vi "IRH3T.vi"(8 "Due Dates":u16[](array[numeric]), 9 "Initial Tardiness":i32, 10 "Schedule 2B Improved":u16[](array[numeric]), 11 "Proocessing Times  (Machines x Jobs)":u16[][](array[numeric])=[[208, 80, 8, 184, 218, 197, 100, 5], [64, 30, 39, 91, 257, 38, 34, 447], [23, 215, 125, 135, 165, 136, 164, 37], [88, 22, 207, 5, 58, 213, 52, 355], [6, 181, 111, 222, 27, 259, 91, 103], [149, 37, 22, 14, 71, 155, 536, 16], [113, 71, 274, 348, 187, 1, 3, 3], [349, 364, 214, 1, 17, 1, 20, 34]]) -> (2 "Total Tardiness":i32, 3 "IRH3T (Reordered) Schedule Out":u16[](array[numeric]))   [LabVIEW 2013]
uses:
  Classes/GanntChart_Class/Operation to Machine Job Tuple.vi
  Classes/GanntChart.lvclass
panel:
  out "IRH3T Schedule Out":u16[](array[numeric])
  out "String":string="Total Tardiness has been improved. Total Tardiness is now %d"
  out "Job Completion Times":u16[](array[numeric])
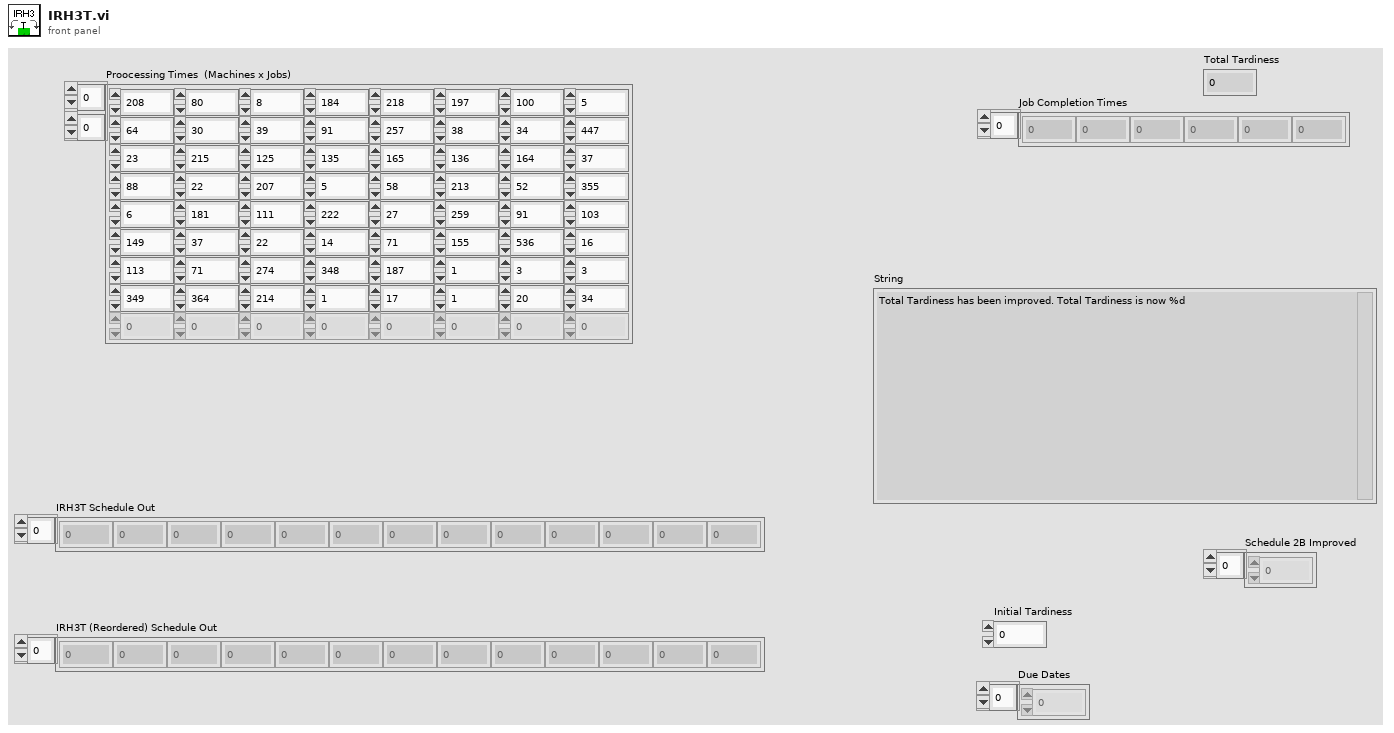
[diagram p1: front panel]
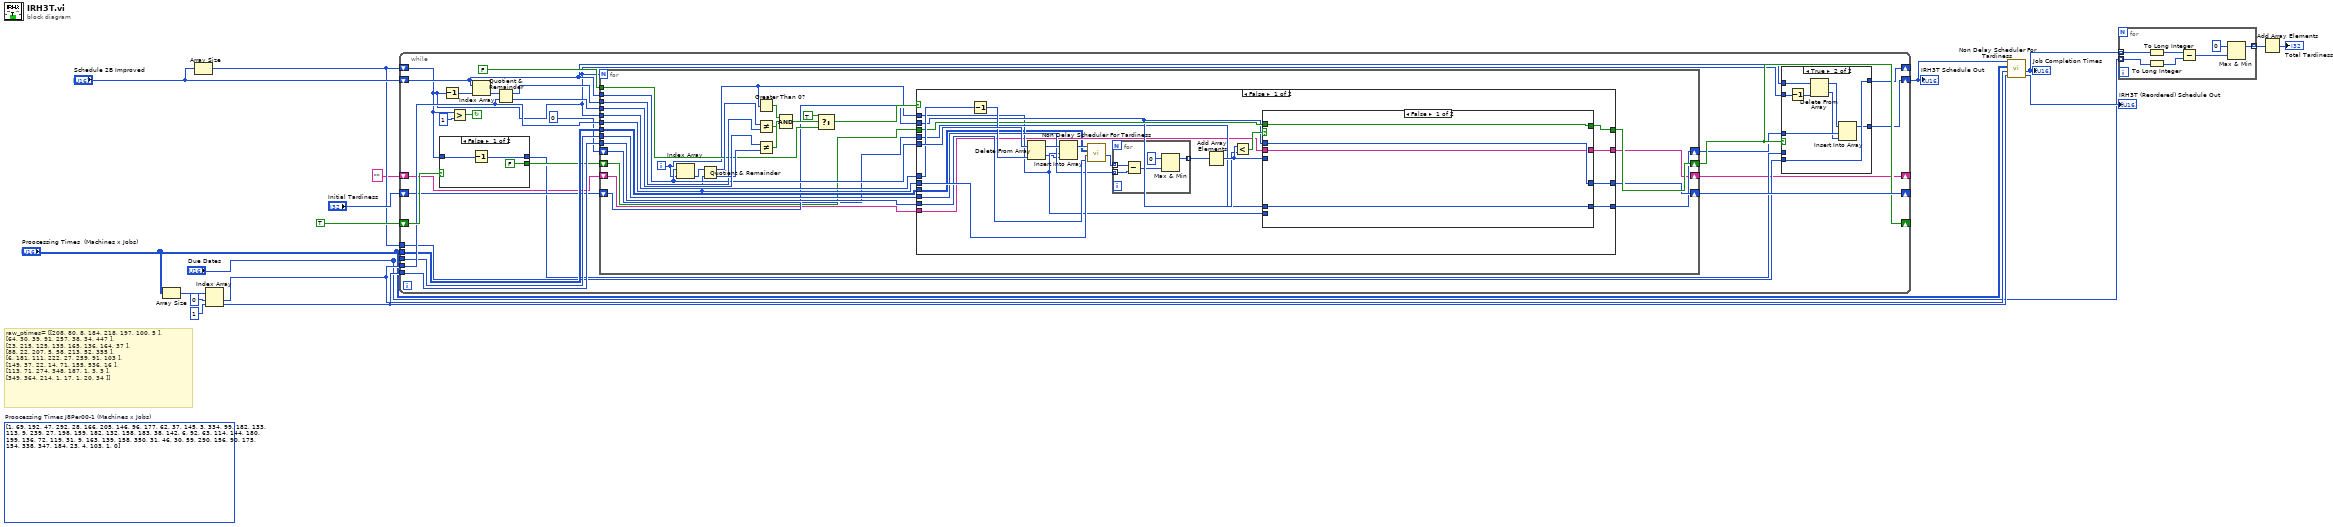
[diagram p0: block diagram]
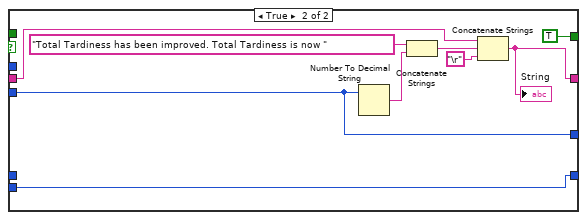
[diagram p3: hidden frame]
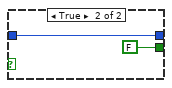
[diagram p5: hidden frame]
diagram:
  (unwired) u16[][] [[1, 69, 192, 47, 292, 28, 166, 205], [146, 96, 177, 62, 37, 145, 3, 334], [99, 182, 133, 113, 9, 239, 27, 198], [159, 182, 132, 158, 183, 38, 142, 6], [92, 63, 114, 144, 180, 199, 136, 72], [119, 31, 9, 163, 139, 158, 350, 31], [46, 30, 59, 290, 156, 90, 175, 154], [338, 347, 184, 23, 4, 103, 1, 0]]  # Proocessing Times J8Per00-1 (Machines x Jobs)
  # "raw_ptimes= [[208, 80, 8, 184, 218, 197, 100, 5 ],\n[64, 30, 39, 91, 257, 38, 34, 447 ],\n[23, 215, 125, 135, 165, 136, 164, 37 ],\n[88, 22, 207, 5, 58, 213, 52, 355 ],\n[6, 181, 111, 222, 27, 259, 91, 103 ],\n[149, 37, 22, 14, 71, 155, 536, 16 ],\n[113, 71, 274, 348, 187, 1, 3, 3 ],\n[349, 364, 214, 1, 17, 1, 20, 34 ]]"
  n1 = Array Size(array="Proocessing Times  (Machines x Jobs)") -> (size(s)=w14:i32[])
  n2 = Array Size(array="Schedule 2B Improved") -> (size(s)=w11:i32)
  n3 = Index Array(array=w14, index #1=0 ("index"), index #2=1 ("index")) -> (element #1=w9:i32, element #2=w8:i32)
  n4 = while {
    shift-right: [w23] -> _
    shift-left: w11 -> [w21]
    shift-right: [w27] -> _
    shift-left: TRUE -> [w41]
    tunnel: w9 -> [w37]
    tunnel: "Proocessing Times  (Machines x Jobs)" -> [w34]
    tunnel: w8 -> [w33]
    tunnel: "Due Dates" -> [w32]
    shift-right: [w29] -> _
    shift-left: "Initial Tardiness" -> [w31]
    shift-right: [w20] -> w10
    shift-left: "Schedule 2B Improved" -> [w26]
    tunnel: w11 -> [w24]
    shift-right: [w18] -> _
    shift-left: "" -> [w19]
    stop <- w42 continue-if-true
    n5 = case shown="False" w41 {
      tunnel: w21 -> [w128 w130]
      tunnel: [w127 w130] -> w22
      tunnel: [FALSE FALSE] -> w30
      frame False {
        n6 = Decrement(x=w128) -> (x-1=w127:i32)
      }
      frame True {
      }
    }
    n7 = Decrement(x=w21) -> (x-1=w40:i32)
    n8 = Greater?(x=w21, y=1) -> (0:w42:bool)
    n9 = Index Array(array=w26, index=w40) -> (element=w39:u16)
    n10 = Quotient & Remainder(x=w39, y=w37) -> (x-y*floor(x/y)=w36:i32, floor(x/y)=w35:i32)
    n11 = for {
      N: w21 -> [_]
      tunnel: FALSE -> [w71]
      tunnel: w26 -> [w68]
      tunnel: w37 -> [w64]
      tunnel: w36 -> [w74]
      tunnel: w35 -> [w78]
      tunnel: w21 -> [w67]
      tunnel: w34 -> [w65]
      tunnel: w33 -> [w63]
      tunnel: w32 -> [w62]
      shift-right: [w59] -> w27
      shift-left: w30 -> [w60]
      shift-right: [w58] -> w29
      shift-left: w31 -> [w61]
      shift-right: [w56] -> w25
      shift-left: 0 -> [w57]
      shift-right: [w54] -> w18
      shift-left: w19 -> [w55]
      i -> [w66]
      n12 = Index Array(array=w68, index=w66) -> (element=w80:u16)
      n13 = Quotient & Remainder(x=w80, y=w64) -> (x-y*floor(x/y)=w75:i32, floor(x/y)=w77:i32)
      n14 = Greater Than 0?(x=w66) -> (x > 0?=w79:bool)
      n15 = Not Equal?(x=w75, y=w74) -> (x != y?=w73:bool)
      n16 = Not Equal?(x=w78, y=w77) -> (x != y?=w76:bool)
      n17 = Compound Arithmetic op=AND(w79, w76, w73) -> (w72:bool)
      n18 = Select(t=TRUE, s=w72, f=w71) -> (s? t:f=w69:bool)
      n19 = case shown="False" w69 {
        tunnel: w68 -> [w103 _]
        tunnel: w67 -> [w102 _]
        tunnel: w66 -> [w85 _]
        tunnel: w65 -> [w82 _]
        tunnel: w64 -> [w98 _]
        tunnel: w63 -> [w97 _]
        tunnel: w62 -> [w94 _]
        tunnel: w61 -> [w88 w124]
        tunnel: w60 -> [w92 w125]
        tunnel: [w91 w125] -> w59
        tunnel: [w89 w124] -> w58
        tunnel: w57 -> [w87 w123]
        tunnel: [w86 w123] -> w56
        tunnel: w55 -> [w84 w122]
        tunnel: [w83 w122] -> w54
        frame False {
          n20 = Decrement(x=w102) -> (x-1=w101:i32)
          n21 = Delete From Array(array=w103, index=w101) -> (deleted portion=w81:u16, array with subset deleted=w100:u16[])  [unwired: 1 in]
          n22 = Insert Into Array(array=w100, index=w85, new element=w81) -> (w99:u16[])
          n23 = call "Non Delay Scheduler For Tardiness.vi"("Number of  Jobs"=w97, "Number of Machines"=w98, "Processing Times"=w82, "Schedule"=w99) -> ("Job Completion Times"=w95:u16[])  [unwired: 3 in, 4 out]
          n24 = for {
            tunnel: w95 -> [w121] mode=indexing
            tunnel: w94 -> [w120] mode=indexing
            tunnel: [w117] -> w96 mode=indexing
            n25 = Subtract(x=w121, y=w120) -> (x-y=w119:u16)
            n26 = Max & Min(x=0, y=w119) -> (max(x,y)=w117:i32)  [unwired: 1 out]
          }
          n27 = Add Array Elements(numeric array=w96) -> (sum=w90:i32)
          n28 = Less?(x=w90, y=w88) -> (x < y?=w93:bool)
          n29 = case shown="False" w93 {
            tunnel: [w107 TRUE] -> w91
            tunnel: w92 -> [w107 _]
            tunnel: w90 -> [_ w114]
            tunnel: [w106 w114] -> w89
            tunnel: w88 -> [w106 _]
            tunnel: w87 -> [w105 _]
            tunnel: [w105 w115] -> w86
            tunnel: w85 -> [_ w115]
            tunnel: w84 -> [w104 w111]
            tunnel: [w104 w108] -> w83
            frame False {
            }
            frame True {
              n30 = Number To Decimal String(number=w114) -> (decimal integer string=w113:string)  [unwired: 1 in]
              n31 = Concatenate Strings("Total Tardiness has been improved. Total Tardiness is now ", w113) -> (w110:string)
              n32 = Concatenate Strings(w111, w110, "\r") -> (w108:string)
              "String" <- w108
            }
          }
        }
        frame True {
        }
      }
    }
    n33 = case shown="True" w27 {
      tunnel: w26 -> [w44 w53]
      tunnel: w21 -> [_ w51]
      tunnel: w25 -> [_ w49]
      tunnel: [w45 w47] -> w23
      tunnel: w24 -> [_ w47]
      tunnel: w22 -> [w45 _]
      tunnel: [w44 w46] -> w20
      frame False {
      }
      frame True {
        n34 = Decrement(x=w51) -> (x-1=w52:i32)
        n35 = Delete From Array(array=w53, index=w52) -> (deleted portion=w48:u16, array with subset deleted=w50:u16[])  [unwired: 1 in]
        n36 = Insert Into Array(array=w50, index=w49, new element=w48) -> (w46:u16[])
      }
    }
  }
  "IRH3T Schedule Out" <- w10
  n37 = call "Non Delay Scheduler For Tardiness.vi"("Number of  Jobs"=w8, "Number of Machines"=w9, "Processing Times"="Proocessing Times  (Machines x Jobs)", "Schedule"=w10) -> ("Scheduled Jobs Order"=→"IRH3T (Reordered) Schedule Out":u16[], "Job Completion Times"=w7:u16[])  [unwired: 3 in, 3 out]
  "Job Completion Times" <- w7
  n38 = for {
    tunnel: w7 -> [w134] mode=indexing
    tunnel: "Due Dates" -> [w133] mode=indexing
    tunnel: [w135] -> w6 mode=indexing
    n39 = To Long Integer(number=w134) -> (32bit integer=w131:i32)
    n40 = To Long Integer(number=w133) -> (32bit integer=w132:i32)
    n41 = Subtract(x=w131, y=w132) -> (x-y=w137:i32)
    n42 = Max & Min(x=0, y=w137) -> (max(x,y)=w135:i32)  [unwired: 1 out]
  }
  n43 = Add Array Elements(numeric array=w6) -> (sum=→"Total Tardiness":i32)
